vi "开门解析.vi"(11 "输入字符串":string="DoorStatus:\nm001-1号,打开,1\n\n[2021-08-02 15:36:06.554]# RECV ASCII>\nRec: 07740e0e000001b70100000000000000022BD67C1E100000\nReasonNo: 44\n卡号: 19047235\n工号: \n姓名: \n部门: \n时间: 2021-08-03 16:03:45 星期二\n地点: m001-1号\n状态: 超级密码开门\n\nRec: 07740e0e000001b80800000000000000022BD67C1A000000\nReasonNo: 23\n时间: 2021-08-02 15:38:45 星期一\n地点: m001-1号\n状态: 门打开[门磁信号]\n\nDoorStatus:\nm001-1号,关闭,2\n\n[2021-08-02 15:36:10.072]# RECV ASCII>\nRec: 07740e0e000001b90900000000000000022BD87C12000000\nReasonNo: 24\n时间: 2021-08-02 15:38:48 星期一\n地点: m001-1号\n状态: 门关闭[门磁信号]\n") -> (3 "门禁输出字符串":string)   [LabVIEW 2016, in "环境动力监测库.lvlib" / "智能门禁监测.lvlib"]
uses:
  <vilib>/regexp/Match Regular Expression.xnode
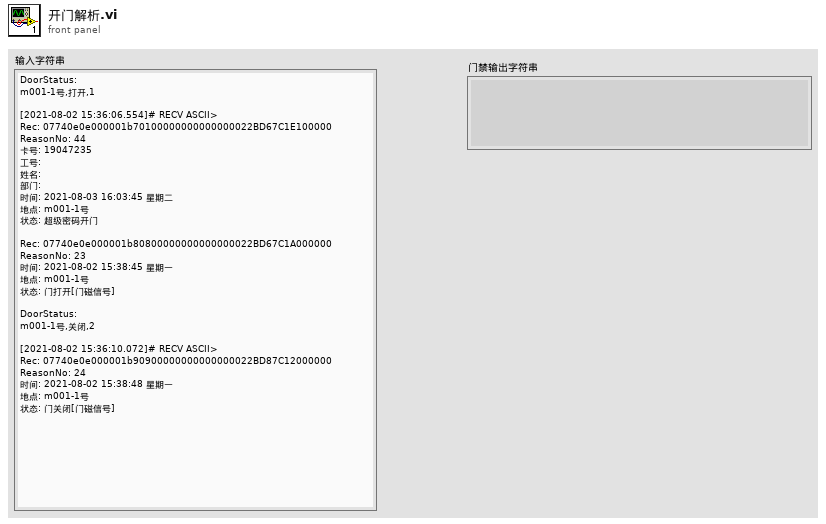
[diagram p1: front panel]
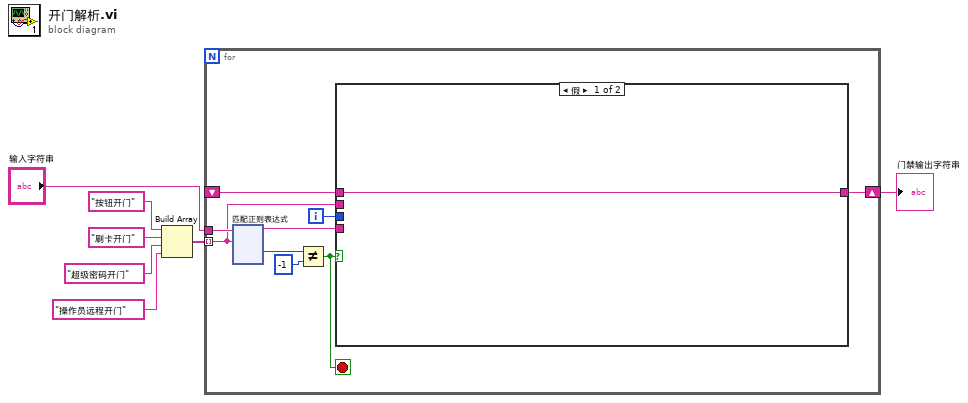
[diagram p0: block diagram]
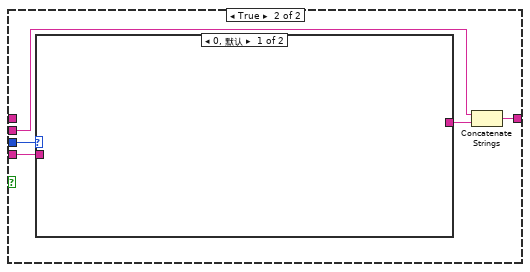
[diagram p2: hidden frame]
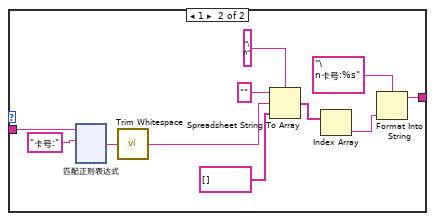
[diagram p3: hidden frame]
diagram:
  n1 = Build Array("按钮开门" ("正则表达式"), "刷卡开门" ("正则表达式"), "超级密码开门" ("正则表达式"), "操作员远程开门" ("正则表达式")) -> (w2:string[])
  n2 = for {
    tunnel: "输入字符串" -> [w16]
    tunnel: w2 -> [w10] mode=indexing
    shift-right: [w9] -> w1
    shift-left: _ -> [w8]
    i -> [w13]
    stop <- w12 stop-if-true
    n3 = xnode "匹配正则表达式"("输入字符串"=w16, "正则表达式"=w10) -> ("匹配之前"=w11:string, "匹配后偏移量"=w15:i32)  [unwired: 4 in, 3 out]
    n4 = Not Equal?(x=w15, y=-1) -> (x != y?=w12:bool)
    n5 = case shown="假" w12 {
      tunnel: w13 -> [_ w22]
      tunnel: w11 -> [_ w21]
      tunnel: w10 -> [_ w18]
      tunnel: [w17 w20] -> w9
      tunnel: w8 -> [w17 _]
      frame False {
      }
      frame True {
        n6 = case shown="0, 默认" w22 {
          tunnel: w21 -> [_ w26]
          tunnel: [_ w23] -> w19
          frame 0, Default {
          }
          frame 1 {
            n7 = xnode "匹配正则表达式"("输入字符串"=w26, "正则表达式"="卡号:") -> ("匹配之后"=w31:string)  [unwired: 4 in, 4 out]
            n8 = call <vilib>:"Trim Whitespace.vi"("string"=w31) -> ("trimmed string"=w32:string)  [unwired: 1 in]
            n9 = Spreadsheet String To Array(delimiter (Tab)="\n" ("分隔符(Tab)"), format string="" ("格式字符串"), spreadsheet string=w32, array type (2D Dbl)=string[] []) -> (array=w33:string[])
            n10 = Index Array(array=w33) -> (element=w24:string)  [unwired: 1 in]
            n11 = Format Into String(format string="\n卡号:%s" ("格式字符串"), w24) -> (resulting string=w23:string)  [unwired: 2 in, 1 out]
          }
        }
        n12 = Concatenate Strings(w18, w19) -> (w20:string)
      }
    }
  }
  "门禁输出字符串" <- w1
